vi "Get Data.vi"(8 "TurnPath?":bool, 11 "Path File":path=path "/home/lvuser/natinst/bin/Paths") -> (0 "V":dbl[](array[numeric]), 1 "Theta":dbl[](array[numeric]), 2 "Path Direction Info":T1, 4 "Command Sequencer Info":T2(array[cluster]), 6 "Initial Angle":dbl)   [LabVIEW 2019]
uses:
  Pathinator/bordeaux-pathinator/Bordeaux/Command Stuff/Single Cmd Info.ctl
  <vilib>/picture/picture.llb/imagedata.ctl
  Pathinator/bordeaux-pathinator/Bordeaux/Limits.ctl
panel:
  out "Path Planner Version":string
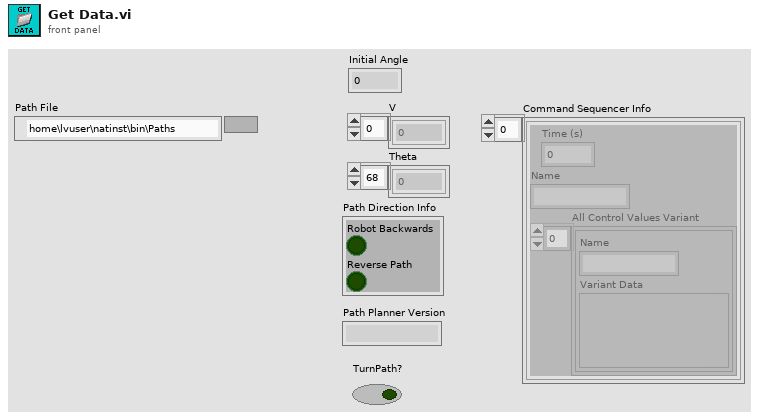
[diagram p1: front panel]
types:
  T1 = cluster{"Robot Backwards":bool, "Reverse Path":bool}
  T2 = cluster{"Time (s)":dbl, "Name":string, "All Control Values Variant":cluster{"Name":string, "Variant Data":variant}[]}[]
  T3 = typedef "Limits.ctl" = cluster{"Velocity (fps)":dbl, "Accel (fps^2)":dbl, "Jerk (fps^3)":dbl, "StoopidFast (fps)":dbl}
  T4 = cluster{"Sample Period (s)":dbl, "Limits":T3, "Conditions":cluster{"vInitial (fps)":dbl, "vFinal (fps)":dbl}, cluster{dbl[], bool[]}}
  T5 = typedef "Single Cmd Info.ctl" = cluster{"Name":string, "CPTM.DataType":variant, "All Control Values Variant":cluster{"Name":string, "Variant Data":variant}[], "icon full":T6, "icon scaled":T6, "Path":path, "Subsystem Color":u32}
  T6 = typedef "imagedata.ctl" = cluster{"image type":i32, "image depth":i32, "image":u8[], "mask":u8[], "colors":u32[], "Rectangle":cluster{"left":i16, "top":i16, "right":i16, "bottom":i16}}
  T7 = cluster{"Segment Name":string, "Type":enum16{"Accel Straight", "Const Straight", "Blend", "Circle"}, "Traj Pos Points":cluster{"x":dbl, "y":dbl, "th":dbl}[], "Traj Vel Points":cluster{"V":dbl, "th":dbl}[], "Accel Index":i32, "Decel Index":i32}[]
  T8 = cluster{"Time (s)":dbl, "Name":string, "All Control Values Variant":cluster{"Name":string, "Variant Data":variant}[]}
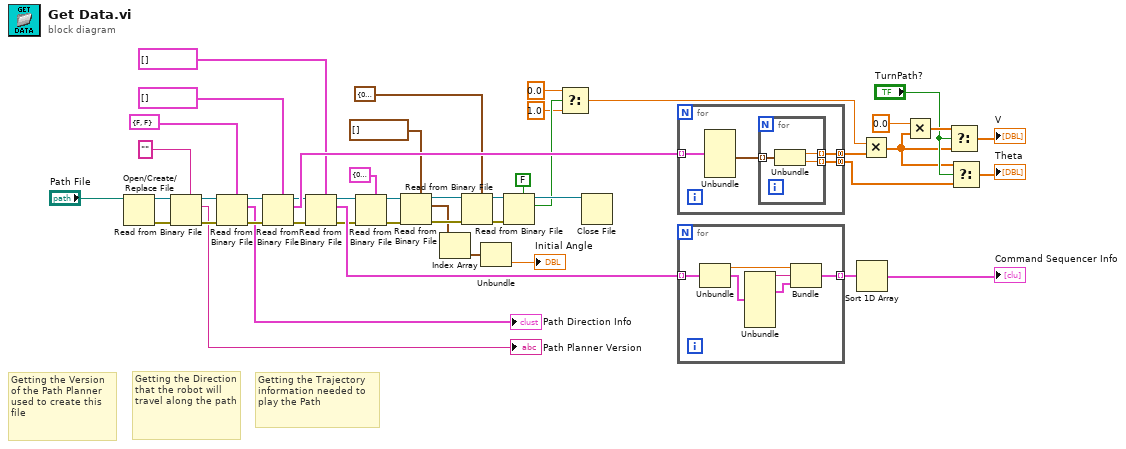
[diagram p0: block diagram]
diagram:
  # "Getting the Trajectory information needed to play the Path"
  # "Getting the Direction that the robot will travel along the path"
  # "Getting the Version of the Path Planner used to create this file"
  n1 = Open/Create/Replace File(file path (use dialog)="Path File") -> (refnum out=w47:refnum<file>, error out=w43:errorcluster)  [unwired: 5 in, 1 out]
  n2 = Read from Binary File(5:"" ("data type"), 8:w43, 11:w47) -> (0:w45:errorcluster, 2:→"Path Planner Version":string, 3:w44:refnum<file>)  [unwired: 3 in, 1 out]
  n3 = Read from Binary File(5:T1 {"Robot Backwards"=FALSE, "Reverse Path"=FALSE} ("output cluster"), 8:w45, 11:w44) -> (0:w42:errorcluster, 2:→"Path Direction Info":T1, 3:w41:refnum<file>)  [unwired: 3 in, 1 out]
  n4 = Read from Binary File(5:T7 [] ("Trajectory Data"), 8:w42, 11:w41) -> (0:w35:errorcluster, 2:w37:T7, 3:w34:refnum<file>)  [unwired: 3 in, 1 out]
  n5 = Read from Binary File(5:cluster{"Time (s)":dbl, T5, bool}[] [], 8:w35, 11:w34) -> (0:w24:errorcluster, 2:w32:cluster{"Time (s)":dbl, T5, bool}[], 3:w27:refnum<file>)  [unwired: 3 in, 1 out]
  n6 = Read from Binary File(5:T4 {"Sample Period (s)"=0.0, "Limits"={"Velocity (fps)"=0.0, "Accel (fps^2)"=0.0, "Jerk (fps^3)"=0.0, "StoopidFast (fps)"=0.0}, "Conditions"={"vInitial (fps)"=0.0, "vFinal (fps)"=0.0}, {[], []}} ("output cluster"), 8:w24, 11:w27) -> (0:w29:errorcluster, 3:w26:refnum<file>)  [unwired: 3 in, 2 out]
  n7 = Read from Binary File(5:cluster{"x":dbl, "y":dbl, "th":dbl}[] [] ("Updated Waypoints"), 8:w29, 11:w26) -> (0:w28:errorcluster, 2:w11:cluster{"x":dbl, "y":dbl, "th":dbl}[], 3:w25:refnum<file>)  [unwired: 3 in, 1 out]
  n8 = Index Array(array=w11) -> (element=w10:cluster{"x":dbl, "y":dbl, "th":dbl})  [unwired: 1 in]
  n9 = Read from Binary File(5:cluster{"Time (s)":dbl, "Distance (ft)":dbl} {"Time (s)"=0.0, "Distance (ft)"=0.0}, 8:w28, 11:w25) -> (0:w23:errorcluster, 3:w22:refnum<file>)  [unwired: 3 in, 2 out]
  n10 = Unbundle(w10) -> ("th"=→"Initial Angle":dbl)  [unwired: 2 out]
  n11 = Read from Binary File(5:FALSE, 8:w23, 11:w22) -> (2:w18:bool, 3:w20:refnum<file>)  [unwired: 3 in, 2 out]
  n12 = Select(t=0.0, s=w18, f=1.0) -> (s? t:f=w15:dbl)
  n13 = Close File(refnum=w20) -> ()  [unwired: 1 in, 2 out]
  n14 = for {
    tunnel: w37 -> [w51] mode=indexing
    tunnel: [w49] -> w19 mode=concatenating
    tunnel: [w48] -> w3 mode=concatenating
    n15 = Unbundle(w51) -> ("Traj Vel Points"=w50:cluster{"V":dbl, "th":dbl}[])  [unwired: 5 out]
    n16 = for {
      tunnel: w50 -> [w54] mode=indexing
      tunnel: [w53] -> w49 mode=indexing
      tunnel: [w52] -> w48 mode=indexing
      n17 = Unbundle(w54) -> ("V"=w53:dbl, "th"=w52:dbl)
    }
  }
  n18 = for {
    tunnel: w32 -> [w60] mode=indexing
    tunnel: [w55] -> w31 mode=indexing
    n19 = Unbundle(w60) -> ("Time (s)"=w58:dbl, w59:T5)  [unwired: 1 out]
    n20 = Unbundle(w59) -> ("Name"=w57:string, "All Control Values Variant"=w56:cluster{"Name":string, "Variant Data":variant}[])  [unwired: 5 out]
    n21 = Bundle("Time (s)"=w58, "Name"=w57, "All Control Values Variant"=w56) -> (w55:T8)  [unwired: 1 in]
  }
  n22 = Sort 1D Array(array=w31) -> (sorted array=→"Command Sequencer Info":T2)
  n23 = Multiply(x=w15, y=w19) -> (x*y=w2:dbl[])
  n24 = Multiply(x=0.0, y=w2) -> (x*y=w6:dbl[])
  n25 = Select(t=w6, s="TurnPath?", f=w2) -> (s? t:f=→"V":dbl[])
  n26 = Select(t=w2, s="TurnPath?", f=w3) -> (s? t:f=→"Theta":dbl[])
